vi "2senser.vi"() -> ()   [LabVIEW 2010]
uses:
  <vilib>/NXT/Block Support/NXT_InputPort.ctl
  <vilib>/NXT/Subs/MotorOutput.ctl
  <vilib>/NXT/Dual Mode Library/Sensors/Light_On.vi
  <vilib>/NXT/Dual Mode Library/Motors/MotorBrake.vi
  <vilib>/NXT/Dual Mode Library/Motors/MotorOn.vi
panel:
  in  "Power (75)":i32=75
  in  "Port (Port 3) 2":T1=2 items=["Port 1", "Port 2", "Port 3", "Port 4"]
  in  "Port (Port 3)":T1=2 items=["Port 1", "Port 2", "Port 3", "Port 4"]
  in  "stop":bool
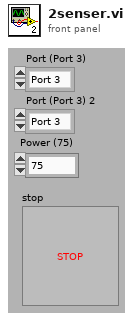
[diagram p1: front panel]
types:
  T1 = typedef "NXT_InputPort.ctl" = u8
  T2 = typedef "MotorOutput.ctl" = u8
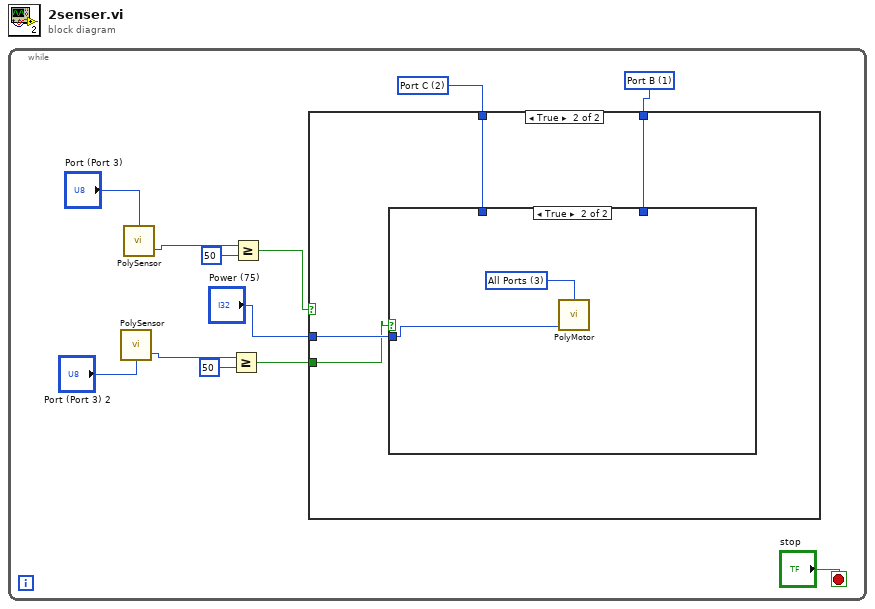
[diagram p0: block diagram]
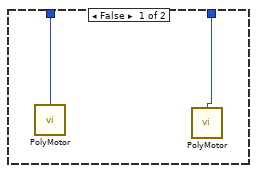
[diagram p3: hidden frame]
diagram:
  n1 = while {
    stop <- "stop" stop-if-true
    w1 = T2 1 items=["Port A", "Port B", "Port C", "All Ports"] ("Output Port (All Ports)")
    w2 = T2 2 items=["Port A", "Port B", "Port C", "All Ports"] ("Output Port (All Ports)")
    n2 = call-poly <vilib>:"PolySensor.vi"("Port (Port 3)"="Port (Port 3) 2") -> ("Scaled Value"=w7:i16)  [unwired: 2 in, 1 out]
    n3 = call-poly <vilib>:"PolySensor.vi"("Port (Port 3)"="Port (Port 3)") -> ("Scaled Value"=w11:i16)  [unwired: 2 in, 1 out]
    n4 = Greater Or Equal?(x=w7, y=i16 50) -> (x >= y?=w3:bool)
    n5 = Greater Or Equal?(x=w11, y=i16 50) -> (x >= y?=w4:bool)
    n6 = case shown="True" w4 {
      tunnel: "Power (75)" -> [_ w16]
      tunnel: w3 -> [_ w15]
      tunnel: w2 -> [_ w14]
      tunnel: w1 -> [_ w13]
      frame False {
      }
      frame True {
        n7 = case shown="True" w15 {
          tunnel: w16 -> [_ w19]
          tunnel: w14 -> [w18 _]
          tunnel: w13 -> [w17 _]
          frame False {
            n8 = call-poly <vilib>:"PolyMotor.vi"("Output Port (All Ports)"=w18) -> ()  [unwired: 3 in, 1 out]
            n9 = call-poly <vilib>:"PolyMotor.vi"("Port (All Ports)"=w17) -> ()  [unwired: 3 in, 1 out]
          }
          frame True {
            w20 = T2 3 items=["Port A", "Port B", "Port C", "All Ports"] ("Output Port (All Ports)")
            n10 = call-poly <vilib>:"PolyMotor.vi"("Power (75)"=w19, "Output Port (All Ports)"=w20) -> ()  [unwired: 2 in, 1 out]
          }
        }
      }
    }
  }
